vi "_Do Delay Time.vi"(0 "DelayTime Address":u16=398) -> ()   [LabVIEW 2012]
uses:
  <vilib>/rvi/Emulation/niFpgaSctlEmulationGetInTimedLoop.vi
  <vilib>/rvi/DataTransferAndStorage/Container/Common/niFpgaContainerGetUniqueNameForEmu.vi
  <vilib>/rvi/Memory/Memory_Emulation/niFpgaMemoryEmulationCacheClearOnFirstRun.vi
  <vilib>/rvi/Memory/Memory_Emulation/nirvimemoryEmulationManagerCache_MakeExclusive.vi
  <vilib>/rvi/Memory/Memory_Emulation/niFpgaMemoryEmulationValidateCache.vi
  <vilib>/rvi/Memory/Memory_Emulation/nirvimemoryEmulationManagerCache_ReleaseExclusive.vi
  <vilib>/rvi/Memory/Memory_Emulation/nirvimemoryEmulationManagerCache_InsertValue.vi
  <vilib>/Utility/error.llb/Clear Errors.vi
  <vilib>/rvi/Memory/Memory_Emulation/nirvimemoryEmulationManagerCache_GetValue.vi
  <vilib>/rvi/DataTransferAndStorage/Container/XNode/niFpgaContainer.xnode
  <vilib>/rvi/Memory/Memory_Emulation/nirvimemoryEmulation.vi
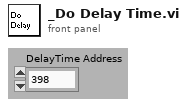
[diagram p1: front panel]
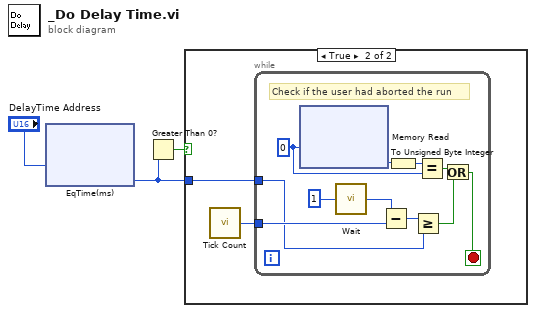
[diagram p0: block diagram]
diagram:
  n1 = xnode ("EqTime(ms)")("Address"="DelayTime Address") -> ("Data"=w3:i16)  [unwired: 1 in, 1 out]
  n2 = Greater Than 0?(x=w3) -> (x > 0?=w2:bool)
  n3 = case shown="True" w2 {
    tunnel: w3 -> [_ w4]
    frame False {
    }
    frame True {
      n4 = call "Tick Count"() -> ("Tick Count(mSec)"=w5:u32)
      n5 = while {
        tunnel: w5 -> [w11]
        tunnel: w4 -> [w9]
        stop <- w6 stop-if-true
        w16 = u8 0 ("Address")
        # "Check if the user had aborted the run"
        n6 = xnode ("Memory Read")("Address"=w16) -> ("Data"=w15:i16)  [unwired: 1 in, 1 out]
        n7 = call "Wait"("Count(mSec)"=u8 1 ("Address")) -> ("Tick Count(mSec)"=w12:u32)
        n8 = Subtract(x=w12, y=w11) -> (x-y=w10:u32)
        n9 = To Unsigned Byte Integer(number=w15) -> (unsigned 8bit integer=w14:u8)
        n10 = Greater Or Equal?(x=w10, y=w9) -> (x >= y?=w8:bool)
        n11 = Equal?(x=w14, y=w16) -> (x = y?=w13:bool)
        n12 = Or(x=w13, y=w8) -> (x .or. y?=w6:bool)
      }
    }
  }
